vi "AO Regs Group UI.vi"(8 "error in (no error)":errorcluster, 11 "Node Ptr":T2 format="%.0x") -> (0 "error out":errorcluster)   [LabVIEW 2020, in "Modbus Master System Explorer.lvlib"]
uses:
  Modbus Master System Explorer.lvlib
  <vilib>/NI VeriStand/Custom Device API/Custom Device Item Ref.ctl
  SubVIs/Conflict Table.ctl
  SubVIs/Modbus Type.ctl
  Shared/Controls/Data Model/Mapping.ctl
  Shared/Controls/Data Model/DataType.ctl
  <vilib>/NI VeriStand/Custom Device API/Custom Device API.lvlib
  <vilib>/NI VeriStand/Custom Device Tools/Custom Device Utility Library/Custom Device Utility Library.lvlib
  Shared/Modbus Master Shared.lvlib
panel:
  in  "Delete Multiple":bool
  in  "Add One":bool
  in  "Bulk Add":bool
  out "Conflicting Holding Register Mappings":T1
  in  "Header":cluster{"Section Name":string}={"Section Name"="Holding Register Group Settings"}
  in  "Description":string
  in  "Name":string
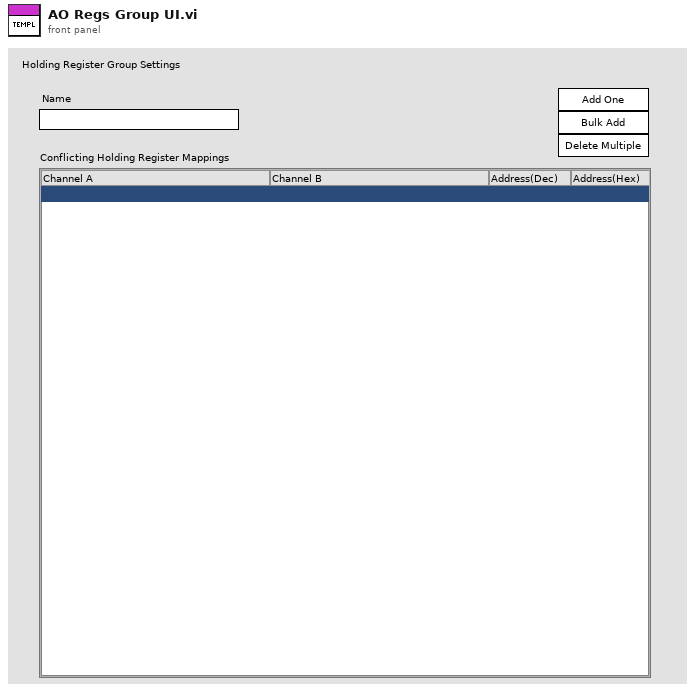
[diagram p1: front panel]
types:
  T1 = typedef "Modbus Master System Explorer.lvlib/Conflict Table.ctl" = i32
  T2 = typedef "Custom Device API.lvlib/Custom Device Item Ref.ctl" = u64
  T3 = typedef "Custom Device API.lvlib/Custom Device Item Info.ctl" = cluster{"Name":string, "Is Channel":bool, "GUID":string, "Is Waveform":bool}
  T4 = cluster{"Name":string, "Name":string, "Mapping":u16}[]
  T5 = typedef "Modbus Master Shared.lvlib/Modbus Type.ctl" = enum16{"Coil", "Discrete Input", "Holding Register", "Input Register"}
  T6 = typedef "Modbus Master Shared.lvlib/Mapping.ctl" = cluster{"DataType":T7, "Starting Address":u16, "Sub-Index (Bool)":u16, "VS Reference":T2}
  T7 = typedef "Modbus Master Shared.lvlib/DataType.ctl" = enum16{"Double", "Single", "I64", "I32", "I16", "I8", "U64", "U32", "U16", "U8", "Boolean"}
  T8 = typedef "Custom Device API.lvlib/Custom Device Commands.ctl" = enum16{"Default", "Item renamed", "Shutdown", "Dynamic button pressed"}
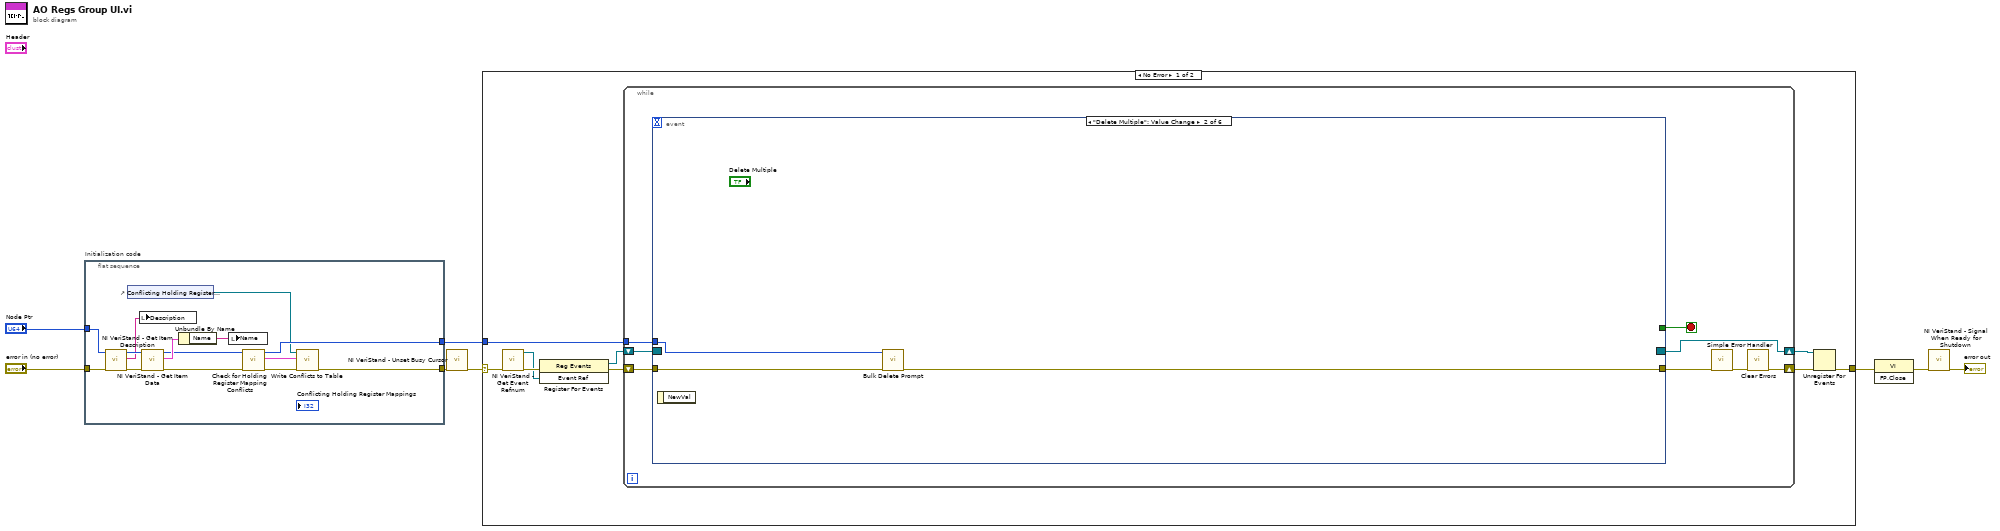
[diagram p0: block diagram]
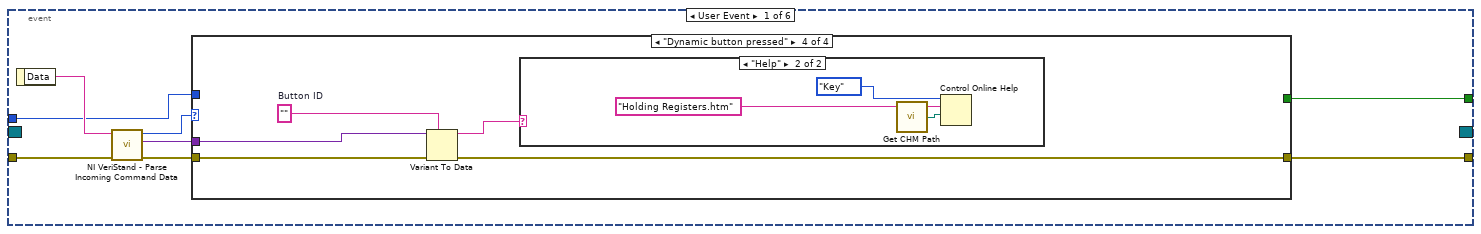
[diagram p2: hidden frame]
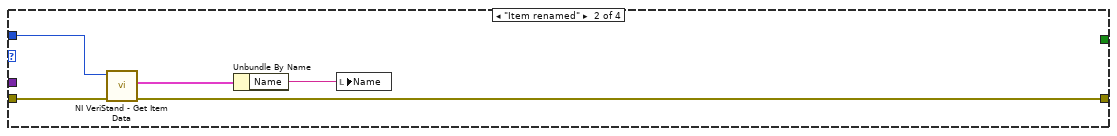
[diagram p4: hidden frame]
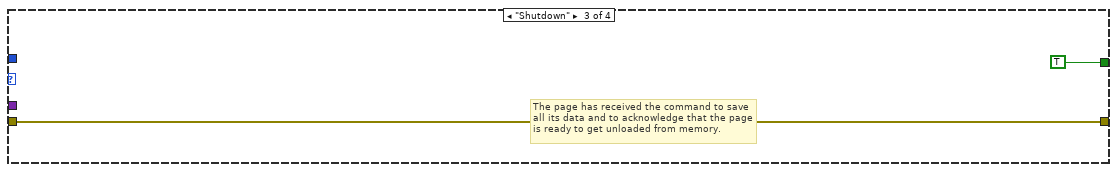
[diagram p5: hidden frame]
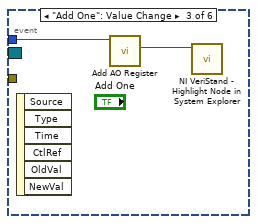
[diagram p7: hidden frame]
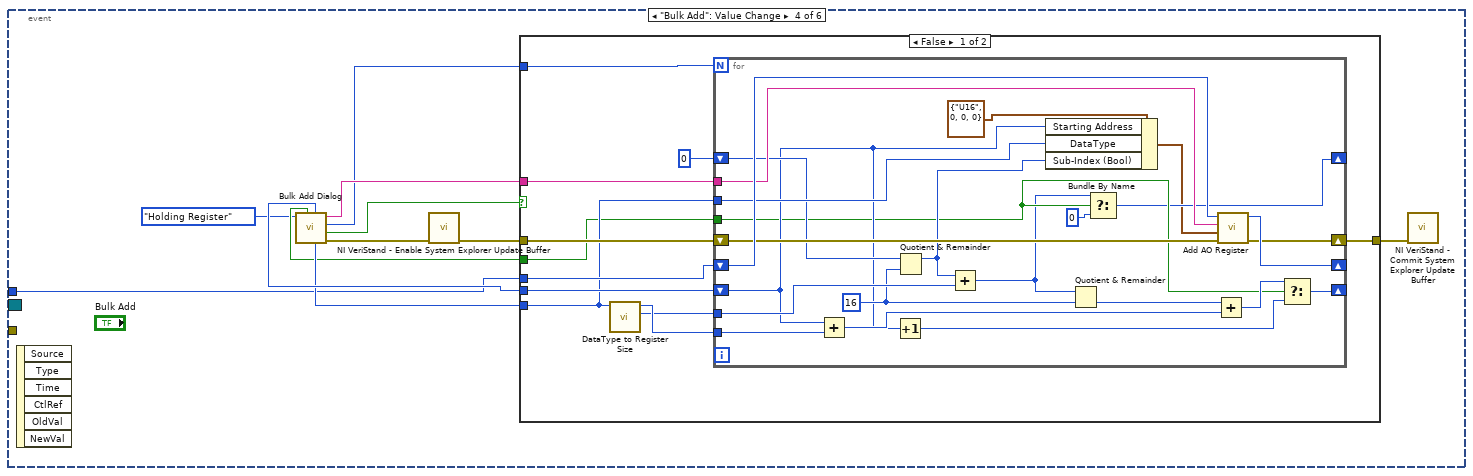
[diagram p8: hidden frame]
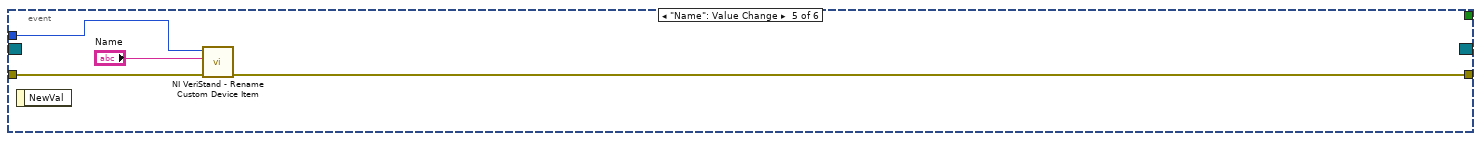
[diagram p10: hidden frame]
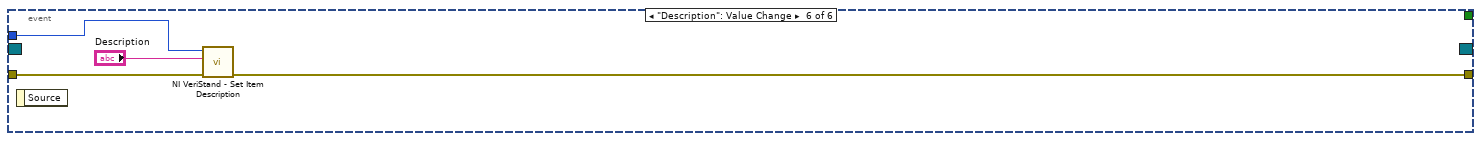
[diagram p11: hidden frame]
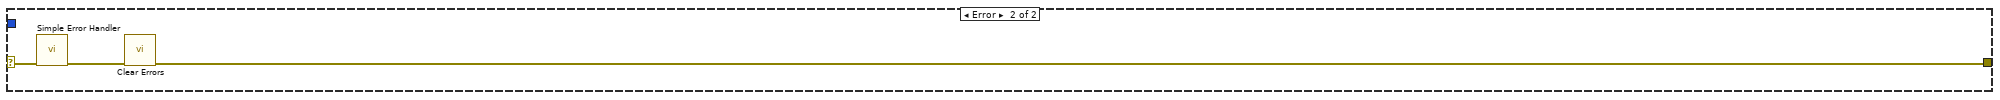
[diagram p12: hidden frame]
diagram:
  n1 = flat-sequence "Initialization code" {
    tunnel: "error in (no error)" -> [w21]
    tunnel: "Node Ptr" -> [w20]
    tunnel: [w12] -> w4
    tunnel: [w14] -> w1
    frame #0 {
      n2 = call <vilib>:"NI VeriStand - Get Item Description.vi"("error in (no error)"=w21, "Item Ref in"=w20) -> ("error out"=w18:errorcluster, "Description"=w19:string, "Item Ref out"=w22:T2)  [unwired: 7 out]
      n3 = control-ref of="Conflicting Holding Register Mappings"() -> (w9:refnum<vi>)
      n4 = local write "Description"(w19) -> ()
      n5 = call <vilib>:"NI VeriStand - Get Item Data.vi"("error in (no error)"=w18, "Item Ref in"=w22) -> ("error out"=w13:errorcluster, "Item Info"=w17:T3, "Item Ref out"=w15:T2)  [unwired: 7 out]
      n6 = Unbundle By Name(w17) -> ("Name"=w16:string)
      n7 = local write "Name"(w16) -> ()
      n8 = call "Check for Holding Register Mapping Conflicts.vi"("error in (no error)"=w13, "Group Ref in"=w15) -> ("error out"=w11:errorcluster, "Conflicts"=w10:T4, "Coil Group Ref out"=w14:T2)  [unwired: 6 in, 1 out]
      n9 = call "Write Conflicts to Table.vi"("error in (no error)"=w11, "Conflicts"=w10, "MC Listbox Ref"=w9) -> ("error out"=w12:errorcluster)  [unwired: 8 in]
    }
  }
  n10 = call <vilib>:"NI VeriStand - Unset Busy Cursor.vi"("error in (no error)"=w4) -> ("error out"=w3:errorcluster)  [unwired: 10 out]
  n11 = case shown="No Error" w3 {
    selector: w3 -> [w23 w125]
    tunnel: [w28 w123] -> w8
    tunnel: w1 -> [w24 _]
    frame No Error {
      n12 = call <vilib>:"NI VeriStand - Get Event Refnum.vi"("error in (no error)"=w23) -> ("error out"=w31:errorcluster, "Event Ref"=w27:refnum<user-event>)  [unwired: 9 out]
      n13 = register-events(error in=w31, w27) -> (reference out=w25:refnum<event-registration>, error out=w26:errorcluster)  [unwired: 1 in]
      n14 = while {
        tunnel: w24 -> [w35]
        shift-right: [w32] -> w29
        shift-left: w26 -> [w38]
        shift-right: [w39] -> w30
        shift-left: w25 -> [w37]
        stop <- w36 stop-if-true
        n15 = event shown="[1] \"Delete Multiple\": Value Change" {
          selector: w37 -> [_ _ _ _ _ _]
          dyn-events: [_ _ _ _ _ _] -> w39
          timeout: _ -> [_ _ _ _ _ _]
          tunnel: w38 -> [w47 w65 _ _ w118 w121]
          tunnel: [w43 _ _ _ _ _] -> w36
          tunnel: [w42 w64 _ _ w117 w120] -> w34
          tunnel: w35 -> [w41 w66 w67 w69 w116 w122]
          event User Event {
            n16 = event-data() -> ("Data"=w46:string)  [unwired: 1 out]
            n17 = call <vilib>:"NI VeriStand - Parse Incoming Command Data.vi"("error in (no error)"=w47, "Incoming data"=w46) -> ("error out"=w45:errorcluster, "Outgoing data"=w40:variant, "Action"=w44:T8)  [unwired: 7 out]
            n18 = case shown="\"Dynamic button pressed\"" w44 {
              tunnel: w45 -> [w48 w53 w54 w60]
              tunnel: [_ _ TRUE _] -> w43
              tunnel: [w48 w50 w54 w57] -> w42
              tunnel: w41 -> [_ w52 _ _]
              tunnel: w40 -> [_ _ _ w59]
              frame "Default", Default {
              }
              frame "Item renamed" {
                n19 = call <vilib>:"NI VeriStand - Get Item Data.vi"("error in (no error)"=w53, "Item Ref in"=w52) -> ("error out"=w50:errorcluster, "Item Info"=w51:T3)  [unwired: 8 out]
                n20 = Unbundle By Name(w51) -> ("Name"=w49:string)
                n21 = local write "Name"(w49) -> ()
              }
              frame "Shutdown" {
                # "The page has received the command to save all its data and to acknowledge that the page is ready to get unloaded from memory."
              }
              frame "Dynamic button pressed" {
                w58 = ""  # Button ID
                n22 = Variant To Data(error in=w60, type=w58, Variant=w59) -> (data=w56:string, error out=w57:errorcluster)
                n23 = case shown="\"Help\"" w56 {
                  frame Default {
                  }
                  frame "Help" {
                    n24 = call "Get CHM Path.vi"() -> ("appended path"=w63:path)
                    n25 = Control Online Help(2:w63, 3:"Holding Registers.htm" ("String to search for"), 4:enum16{"Contents", "Key", "Close"}."Key" ("Operation")) -> ()  [unwired: 1 in, 1 out]
                  }
                }
              }
            }
          }
          event "Delete Multiple": Value Change {
            n26 = event-data() -> ()  [unwired: 2 out]
            n27 = call "Bulk Delete Prompt.vi"("error in (no error)"=w65, "Item Ref in"=w66) -> ("error out"=w64:errorcluster)  [unwired: 9 in]
          }
          event "Add One": Value Change {
            n28 = event-data() -> ()  [unwired: 7 out]
            n29 = call "Add AO Register.vi"("Node Ref In"=w67) -> ("Channel Ref out"=w68:T2)  [unwired: 8 in, 2 out]
            n30 = call <vilib>:"NI VeriStand - Highlight Node in System Explorer.vi"("Item Ref in"=w68) -> ()  [unwired: 9 in, 2 out]
          }
          event "Bulk Add": Value Change {
            n31 = event-data() -> ()  [unwired: 7 out]
            n32 = call "Bulk Add Dialog.vi"("Type"=Modbus_Type."Holding Register") -> ("error out"=w73:errorcluster, "Cancelled?"=w76:bool, "Quantity Out"=w77:u16, "Root Name Out"=w78:string, "DataType Out"=w75:T7, "Starting Address Out"=w79:u16, "Pack Values? Out"=w74:bool)  [unwired: 4 in]
            n33 = call <vilib>:"NI VeriStand - Enable System Explorer Update Buffer.vi"("error in (no error)"=w73) -> ("error out"=w72:errorcluster)  [unwired: 10 in]
            n34 = case shown="False" w76 {
              tunnel: w69 -> [w83 _]
              tunnel: w77 -> [w90 _]
              tunnel: w72 -> [w84 w114]
              tunnel: w78 -> [w89 _]
              tunnel: w79 -> [w88 _]
              tunnel: w75 -> [w82 _]
              tunnel: w74 -> [w81 _]
              tunnel: [w80 w114] -> w71
              frame False {
                n35 = call "DataType to Register Size.vi"("DataType"=w82) -> ("bits"=w85:i32, "Registers"=w87:i32)  [unwired: 9 in]
                n36 = for {
                  N: w90 -> [_]
                  shift-right: [w111] -> _
                  shift-left: w83 -> [w113]
                  shift-right: [w109] -> w80
                  shift-left: w84 -> [w112]
                  tunnel: w89 -> [w110]
                  shift-right: [w96] -> _
                  shift-left: w88 -> [w98]
                  tunnel: w82 -> [w107]
                  tunnel: w87 -> [w106]
                  shift-right: [w93] -> _
                  shift-left: 0 ("Sub-Index (Bool)") -> [w104]
                  tunnel: w85 -> [w105]
                  tunnel: w81 -> [w95]
                  w101 = 16 ("y")
                  n37 = Add(x=w98, y=w106) -> (x+y=w102:i32)
                  n38 = Increment(x=w98) -> (x+1=w99:i32)
                  n39 = Quotient & Remainder(x=w104, y=w101) -> (x-y*floor(x/y)=w103:i32)  [unwired: 1 out]
                  n40 = Add(x=w103, y=w105) -> (x+y=w94:i32)
                  n41 = Bundle By Name(cluster=T6 {"DataType"=enum."U16", "Starting Address"=0, "Sub-Index (Bool)"=0, "VS Reference"=0} ("Mapping"), "Starting Address"=w98, "DataType"=w107, "Sub-Index (Bool)"=w103) -> (w91:T6)
                  n42 = Quotient & Remainder(x=w94, y=w101) -> (floor(x/y)=w100:i32)  [unwired: 1 out]
                  n43 = Select(t=w94, s=w95, f=0 ("t")) -> (s? t:f=w93:i32)
                  n44 = Add(x=w100, y=w102) -> (x+y=w97:i32)
                  n45 = call "Add AO Register.vi"("error in (no error)"=w112, "Mapping"=w91, "Label"=w110, "Node Ref In"=w113) -> ("error out"=w109:errorcluster, "Node Ref out"=w111:T2)  [unwired: 5 in, 1 out]
                  n46 = Select(t=w97, s=w95, f=w99) -> (s? t:f=w96:i32)
                }
              }
              frame True {
              }
            }
            n47 = call <vilib>:"NI VeriStand - Commit System Explorer Update Buffer.vi"("error in (no error)"=w71) -> ()  [unwired: 10 in, 1 out]
          }
          event "Name": Value Change {
            n48 = event-data() -> ()  [unwired: 2 out]
            n49 = call <vilib>:"NI VeriStand - Rename Custom Device Item.vi"("error in (no error)"=w118, "New Name"="Name", "Item Ref in"=w116) -> ("error out"=w117:errorcluster)  [unwired: 1 in, 7 out]
          }
          event "Description": Value Change {
            n50 = event-data() -> ()  [unwired: 2 out]
            n51 = call <vilib>:"NI VeriStand - Set Item Description.vi"("error in (no error)"=w121, "Description"="Description", "Item Ref in"=w122) -> ("error out"=w120:errorcluster)  [unwired: 8 out]
          }
        }
        n52 = call <vilib>:"Simple Error Handler.vi"("error in (no error)"=w34) -> ("error out"=w33:errorcluster)  [unwired: 1 in, 7 out]
        n53 = call <vilib>:"Clear Errors.vi"("error in (no error)"=w33) -> ("error out"=w32:errorcluster)  [unwired: 1 in, 5 out]
      }
      n54 = Unregister For Events(event registration refnum=w30, error in=w29) -> (error out=w28:errorcluster)
    }
    frame Error {
      n55 = call <vilib>:"Simple Error Handler.vi"("error in (no error)"=w125) -> ("error out"=w124:errorcluster)  [unwired: 1 in, 7 out]
      n56 = call <vilib>:"Clear Errors.vi"("error in (no error)"=w124) -> ("error out"=w123:errorcluster)  [unwired: 1 in, 5 out]
    }
  }
  n57 = invoke class="VI" method="FP.Close"(error in=w8) -> (error out=w7:errorcluster)  [unwired: 2 in, 2 out]
  n58 = call <vilib>:"NI VeriStand - Signal When Ready for Shutdown.vi"("error in (no error)"=w7) -> ("error out"=→"error out":errorcluster)  [unwired: 10 out]
